vi "OCUtoSim.vi"() -> ()   [LabVIEW 2011]
uses:
  2-Think/2 Typedefs/UTM Location.ctl
panel:
  in  "Robot UTM Location":T1 {"North" format="%#_10f"; "East" format="%#_8f"}
  in  "Move boat?":bool
  in  "Boat Heading":dbl
  in  "Pause Simulator?":bool
  in  "Wind Speed":dbl
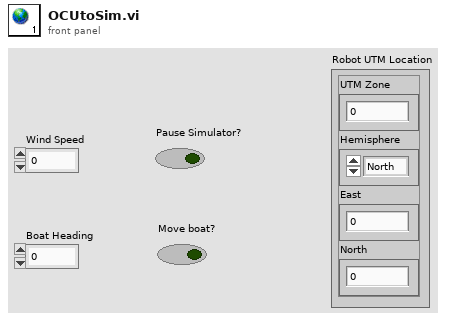
[diagram p1: front panel]
types:
  T1 = typedef "UTM Location.ctl" = cluster{"UTM Zone":dbl, "Hemisphere":enum16{"North", "South"}, "East":dbl, "North":dbl}
diagram:
